vi "RT Driver_Coef and Max Range.vi"(8 "error in (no error)":errorcluster, 11 "Offset (s)":dbl format="%_6p") -> (0 "error out":errorcluster, 1 "output range":cluster{"output high":dbl, "output low":dbl}={"output high"=50.0, "output low"=-50.0}, 2 "index out":i32, 3 "PID gains out":T1, 4 "Reset":bool)   [LabVIEW 2013]
uses:
  <vilib>/addons/control/pid/pid.llb/PID Gain Schedule (DBL).vi
  <vilib>/addons/control/pid/NI_PID_pid.lvlib
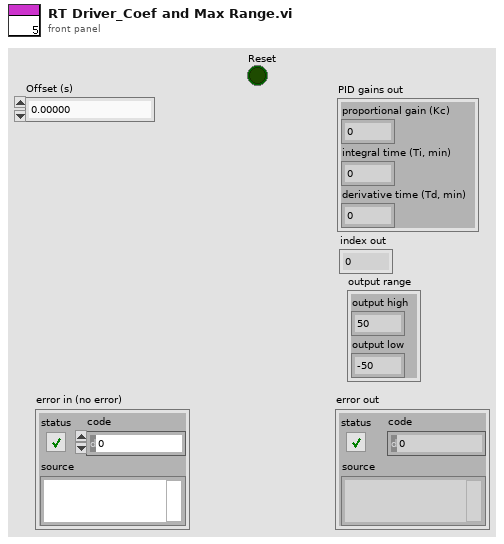
[diagram p1: front panel]
types:
  T1 = cluster{"proportional gain (Kc)":dbl, "integral time (Ti, min)":dbl, "derivative time (Td, min)":dbl}
  T2 = cluster{"PID gains":cluster{"proportional gain (Kc)":dbl, "integral time (Ti, min)":dbl, "derivative time (Td, min)":dbl}, "max value":dbl}[]
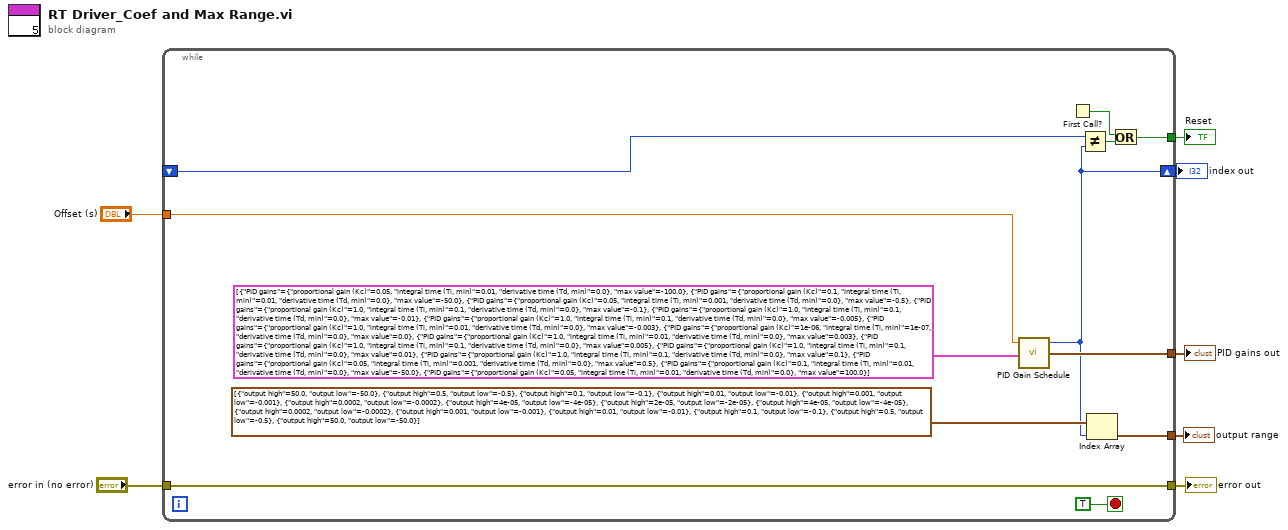
[diagram p0: block diagram]
diagram:
  n1 = while {
    tunnel: [w19] -> w7
    tunnel: "Offset (s)" -> [w17]
    tunnel: [w15] -> w4
    tunnel: "error in (no error)" -> [w13]
    tunnel: [w13] -> w2
    shift-right: [w12] -> w5
    shift-left: _ -> [w11]
    tunnel: [w8] -> w1
    stop <- TRUE stop-if-true
    n2 = call-poly <vilib>:"PID Gain Schedule.vi"("PID gain schedule"=T2 [{"PID gains"={"proportional gain (Kc)"=0.05, "integral time (Ti, min)"=0.01, "derivative time (Td, min)"=0.0}, "max value"=-100.0}, {"PID gains"={"proportional gain (Kc)"=0.1, "integral time (Ti, min)"=0.01, "derivative time (Td, min)"=0.0}, "max value"=-50.0}, {"PID gains"={"proportional gain (Kc)"=0.05, "integral time (Ti, min)"=0.001, "derivative time (Td, min)"=0.0}, "max value"=-0.5}, {"PID gains"={"proportional gain (Kc)"=1.0, "integral time (Ti, min)"=0.1, "derivative time (Td, min)"=0.0}, "max value"=-0.1}, {"PID gains"={"proportional gain (Kc)"=1.0, "integral time (Ti, min)"=0.1, "derivative time (Td, min)"=0.0}, "max value"=-0.01}, {"PID gains"={"proportional gain (Kc)"=1.0, "integral time (Ti, min)"=0.1, "derivative time (Td, min)"=0.0}, "max value"=-0.005}, {"PID gains"={"proportional gain (Kc)"=1.0, "integral time (Ti, min)"=0.01, "derivative time (Td, min)"=0.0}, "max value"=-0.003}, {"PID gains"={"proportional gain (Kc)"=1e-06, "integral time (Ti, min)"=1e-07, "derivative time (Td, min)"=0.0}, "max value"=0.0}, {"PID gains"={"proportional gain (Kc)"=1.0, "integral time (Ti, min)"=0.01, "derivative time (Td, min)"=0.0}, "max value"=0.003}, {"PID gains"={"proportional gain (Kc)"=1.0, "integral time (Ti, min)"=0.1, "derivative time (Td, min)"=0.0}, "max value"=0.005}, {"PID gains"={"proportional gain (Kc)"=1.0, "integral time (Ti, min)"=0.1, "derivative time (Td, min)"=0.0}, "max value"=0.01}, {"PID gains"={"proportional gain (Kc)"=1.0, "integral time (Ti, min)"=0.1, "derivative time (Td, min)"=0.0}, "max value"=0.1}, {"PID gains"={"proportional gain (Kc)"=0.05, "integral time (Ti, min)"=0.001, "derivative time (Td, min)"=0.0}, "max value"=0.5}, {"PID gains"={"proportional gain (Kc)"=0.1, "integral time (Ti, min)"=0.01, "derivative time (Td, min)"=0.0}, "max value"=-50.0}, {"PID gains"={"proportional gain (Kc)"=0.05, "integral time (Ti, min)"=0.01, "derivative time (Td, min)"=0.0}, "max value"=100.0}], "gain scheduling value"=w17) -> ("PID gains out"=w19:T1, "index out"=w12:i32)  [unwired: 2 in]
    n3 = First Call?() -> (First Call?: T/F=w9:bool)
    n4 = Not Equal?(x=w11, y=w12) -> (x != y?=w10:bool)
    n5 = Index Array(array=cluster{"output high":dbl, "output low":dbl}[] [{"output high"=50.0, "output low"=-50.0}, {"output high"=0.5, "output low"=-0.5}, {"output high"=0.1, "output low"=-0.1}, {"output high"=0.01, "output low"=-0.01}, {"output high"=0.001, "output low"=-0.001}, {"output high"=0.0002, "output low"=-0.0002}, {"output high"=4e-05, "output low"=-4e-05}, {"output high"=2e-05, "output low"=-2e-05}, {"output high"=4e-05, "output low"=-4e-05}, {"output high"=0.0002, "output low"=-0.0002}, {"output high"=0.001, "output low"=-0.001}, {"output high"=0.01, "output low"=-0.01}, {"output high"=0.1, "output low"=-0.1}, {"output high"=0.5, "output low"=-0.5}, {"output high"=50.0, "output low"=-50.0}], index=w12) -> (element=w15:cluster{"output high":dbl, "output low":dbl})
    n6 = Or(x=w9, y=w10) -> (x .or. y?=w8:bool)
  }
  "index out" <- w5
  "PID gains out" <- w7
  "error out" <- w2
  "output range" <- w4
  "Reset" <- w1
